vi "Even Ends.vi"(8 "Array":dbl[](array[numeric]), 10 "Odd?":bool, 11 "delta_x":dbl) -> (2 "Trap Value":dbl)   [LabVIEW 2017]
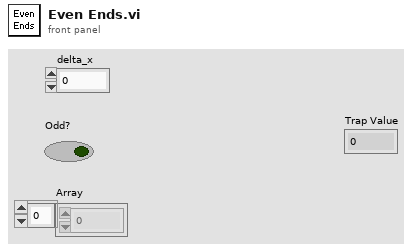
[diagram p1: front panel]
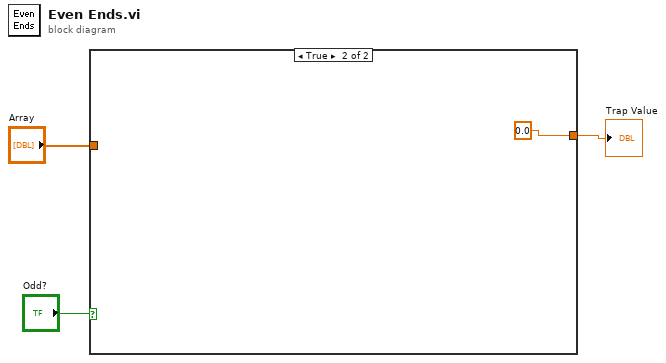
[diagram p0: block diagram]
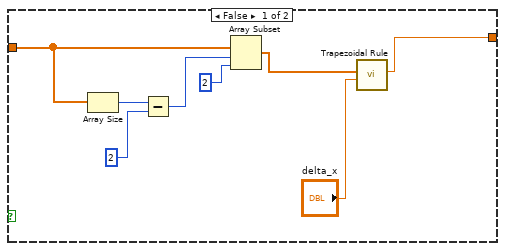
[diagram p2: hidden frame]
diagram:
  n1 = case shown="True" "Odd?" {
    tunnel: "Array" -> [w9 _]
    tunnel: [w4 0.0] -> w1
    frame False {
      n2 = Array Size(array=w9) -> (size(s)=w8:i32)
      n3 = Subtract(x=w8, y=2) -> (x-y=w6:i32)
      n4 = Array Subset(array=w9, index=w6, length=2) -> (w10:dbl[])
      n5 = call "Trapezoidal Rule.vi"("Delta_x"="delta_x", "y array"=w10) -> ("Value of Integral"=w4:dbl)  [unwired: 9 in]
    }
    frame True {
    }
  }
  "Trap Value" <- w1
